vi "cage manager.vi"(7 "Set/Get":T2=enum."Get", 8 "Error In":errorcluster, 9 "Cluster In":T3={"Position"=0.0, "Is.Enabled?"=FALSE, "Is.Connected?"=FALSE, "Device SN"="55151324", "AccelerationMaximum"=0.0, "VelocityMaximum"=0.0, "Acceleration"=0.0, "Velocity"=0.0, "waitTimeout (ms)"=10000, "Model"=enum."None", "Is.Homed?"=FALSE}, 10 "LTS Reference":refnum<k24>(container)) -> (0 "Error Out":errorcluster, 1 "Cluster Out":T3={"Position"=0.0, "Is.Enabled?"=FALSE, "Is.Connected?"=FALSE, "Device SN"="45876539", "AccelerationMaximum"=0.0, "VelocityMaximum"=0.0, "Acceleration"=0.0, "Velocity"=0.0, "waitTimeout (ms)"=0, "Model"=enum."None", "Is.Homed?"=FALSE})   [LabVIEW 2018]
uses:
  C:/Project/SerialSectionOCT/SerialSectOCT/Labview Software/Thorlabs.MotionControl.Controls.dll
  Thorlabs.MotionControl.Controls.dll
  Thorlabs Translation Stages/Controls/Translation Stage Cluster.ctl
  General/Controls/Translation Stage Types.ctl
  General/Controls/Set Get Controls.ctl
  Thorlabs Translation Stages/Controls/Motion Translation Module Control2.ctl
panel:
  in  "Action 4":T1
  in  "Action 3":T1
  in  "Action 2":T1
  in  "Action":T1
  in  "Set/Get 4":T2=enum."Get"
  in  "Set/Get 3":T2=enum."Get"
  in  "Set/Get 2":T2=enum."Get"
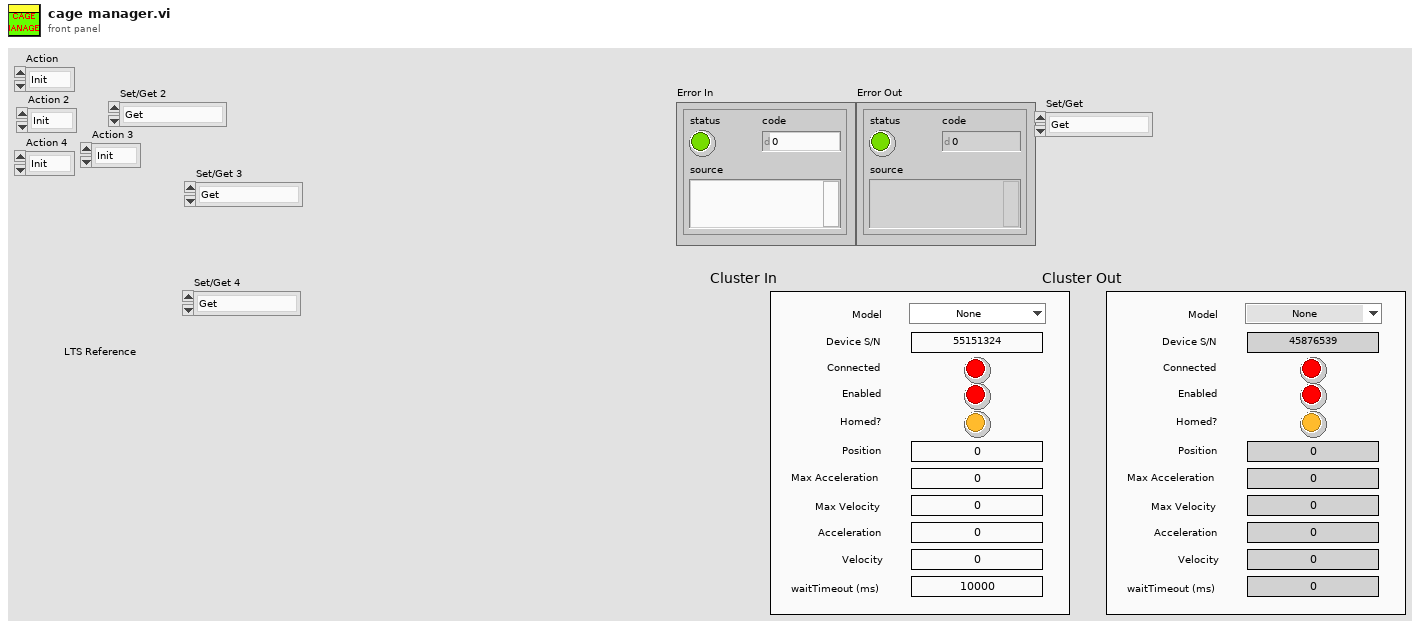
[diagram p1: front panel]
types:
  T1 = typedef "Motion Translation Module Control2.ctl" = enum16{"Init", "Home", "Status", "Velocity/Accel", "Position", "Jog", "Stop", "Uninit", "Enable", "Disable"}
  T2 = typedef "Set Get Controls.ctl" = enum16{"Set", "Get"}
  T3 = typedef "Translation Stage Cluster.ctl" = cluster{"Position":dbl, "Is.Enabled?":bool, "Is.Connected?":bool, "Device SN":string, "AccelerationMaximum":dbl, "VelocityMaximum":dbl, "Acceleration":dbl, "Velocity":dbl, "waitTimeout (ms)":i32, "Model":T4, "Is.Homed?":bool}
  T4 = typedef "Translation Stage Types.ctl" = enum16{"None", "Thorlabs LTS", "Thorlabs MLJ"}
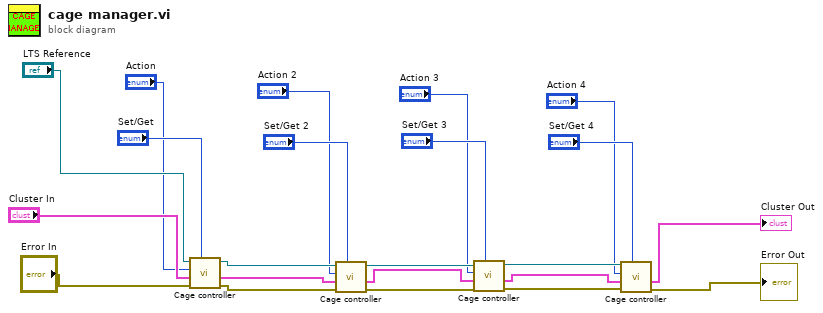
[diagram p0: block diagram]
diagram:
  n1 = call "Cage controller.vi"("Set/Get"="Set/Get", "error in (no error)"="Error In", "Cluster In"="Cluster In", "Action"="Action", "reference in"="LTS Reference") -> ("error out"=w12:errorcluster, "Cluster out"=w9:T3, "reference out"=w15:refnum<k24>)  [unwired: 4 in]
  n2 = call "Cage controller.vi"("Set/Get"="Set/Get 2", "error in (no error)"=w12, "Cluster In"=w9, "Action"="Action 2", "reference in"=w15) -> ("error out"=w11:errorcluster, "Cluster out"=w8:T3, "reference out"=w14:refnum<k24>)  [unwired: 4 in]
  n3 = call "Cage controller.vi"("Set/Get"="Set/Get 3", "error in (no error)"=w11, "Cluster In"=w8, "Action"="Action 3", "reference in"=w14) -> ("error out"=w10:errorcluster, "Cluster out"=w7:T3, "reference out"=w13:refnum<k24>)  [unwired: 4 in]
  n4 = call "Cage controller.vi"("Set/Get"="Set/Get 4", "error in (no error)"=w10, "Cluster In"=w7, "Action"="Action 4", "reference in"=w13) -> ("error out"=→"Error Out":errorcluster, "Cluster out"=→"Cluster Out":T3)  [unwired: 4 in, 1 out]
